vi "Calculate-MSCN x-axis value.vi"(5 "Total number of points in indexed ROI over the full experiment time":i32, 7 "Number of pixels in ROI":i32, 9 "Header Data":T1={"Number of POI"=0, "Number of Miniscans"=0, "Number of Trials"=0, "Number of Cycles "=0, "# Averaged Frames"=0, "Laser power (%)"=0, "Pockels"=0.0, "Acquisition Length (sec)"=0.0, "Fill time (us)"=0.0, "DwellTime (us)"=0.0, "Miniscan Dwell time per pixel (us)"=0.0, "PMT 1"=0.0, "PMT 2"=0.0, "Back Apperture"=0.0, "Zoom"=0.0, "Number of Pixels in Miniscan"=0, "Frame Size"=200, "Field of View"=0.0, "X centre"=0.0, "Y centre"=0.0, "AOL Z"=0.0} {"Frame Size" items=["100X100"=100, "128X128"=128, "200X200"=200, "256X256"=256, "512X512"=512, "1024x1024"=1024, "2048x2048"=2048]; "Back Apperture" format="%#.6g"; "Pockels" format="%#.6g"; "PMT 2" format="%#.6g"; "PMT 1" format="%#.6g"; "Miniscan Dwell time per pixel (us)" format="%#.6g"; "Zoom" format="%#.6g"; "DwellTime (us)" format="%#.6g"; "Acquisition Length (sec)" format="%#.6g"; "Fill time (us)" format="%#.6g"}, 10 "[ROI Time(us)]":dbl[](array[numeric]), 11 "ROI number":i32=1) -> (1 "MSCN X-axis values array (sec)":sgl[](array[numeric]) format="%#.9f")   [LabVIEW 2020]
uses:
  Experiment header interface/Typedefs/Header parameters cluster-Zstack.ctl
  Typedefs/Frame Size.ctl
panel:
  out "Array":i32[](array[numeric])
  # "Zstack header parameters"
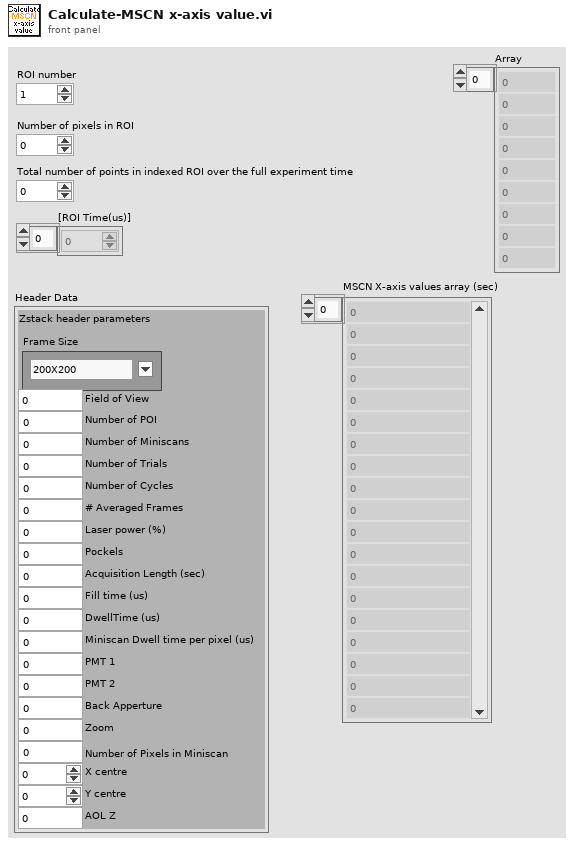
[diagram p1: front panel]
types:
  T1 = typedef "Header parameters cluster-Zstack.ctl" = cluster{"Number of POI":u16, "Number of Miniscans":u16, "Number of Trials":u16, "Number of Cycles ":u16, "# Averaged Frames":u16, "Laser power (%)":u8, "Pockels":dbl, "Acquisition Length (sec)":dbl, "Fill time (us)":dbl, "DwellTime (us)":dbl, "Miniscan Dwell time per pixel (us)":dbl, "PMT 1":dbl, "PMT 2":dbl, "Back Apperture":dbl, "Zoom":dbl, "Number of Pixels in Miniscan":u16, "Frame Size":T2, "Field of View":dbl, "X centre":dbl, "Y centre":dbl, "AOL Z":dbl}
  T2 = typedef "Frame Size.ctl" = u16
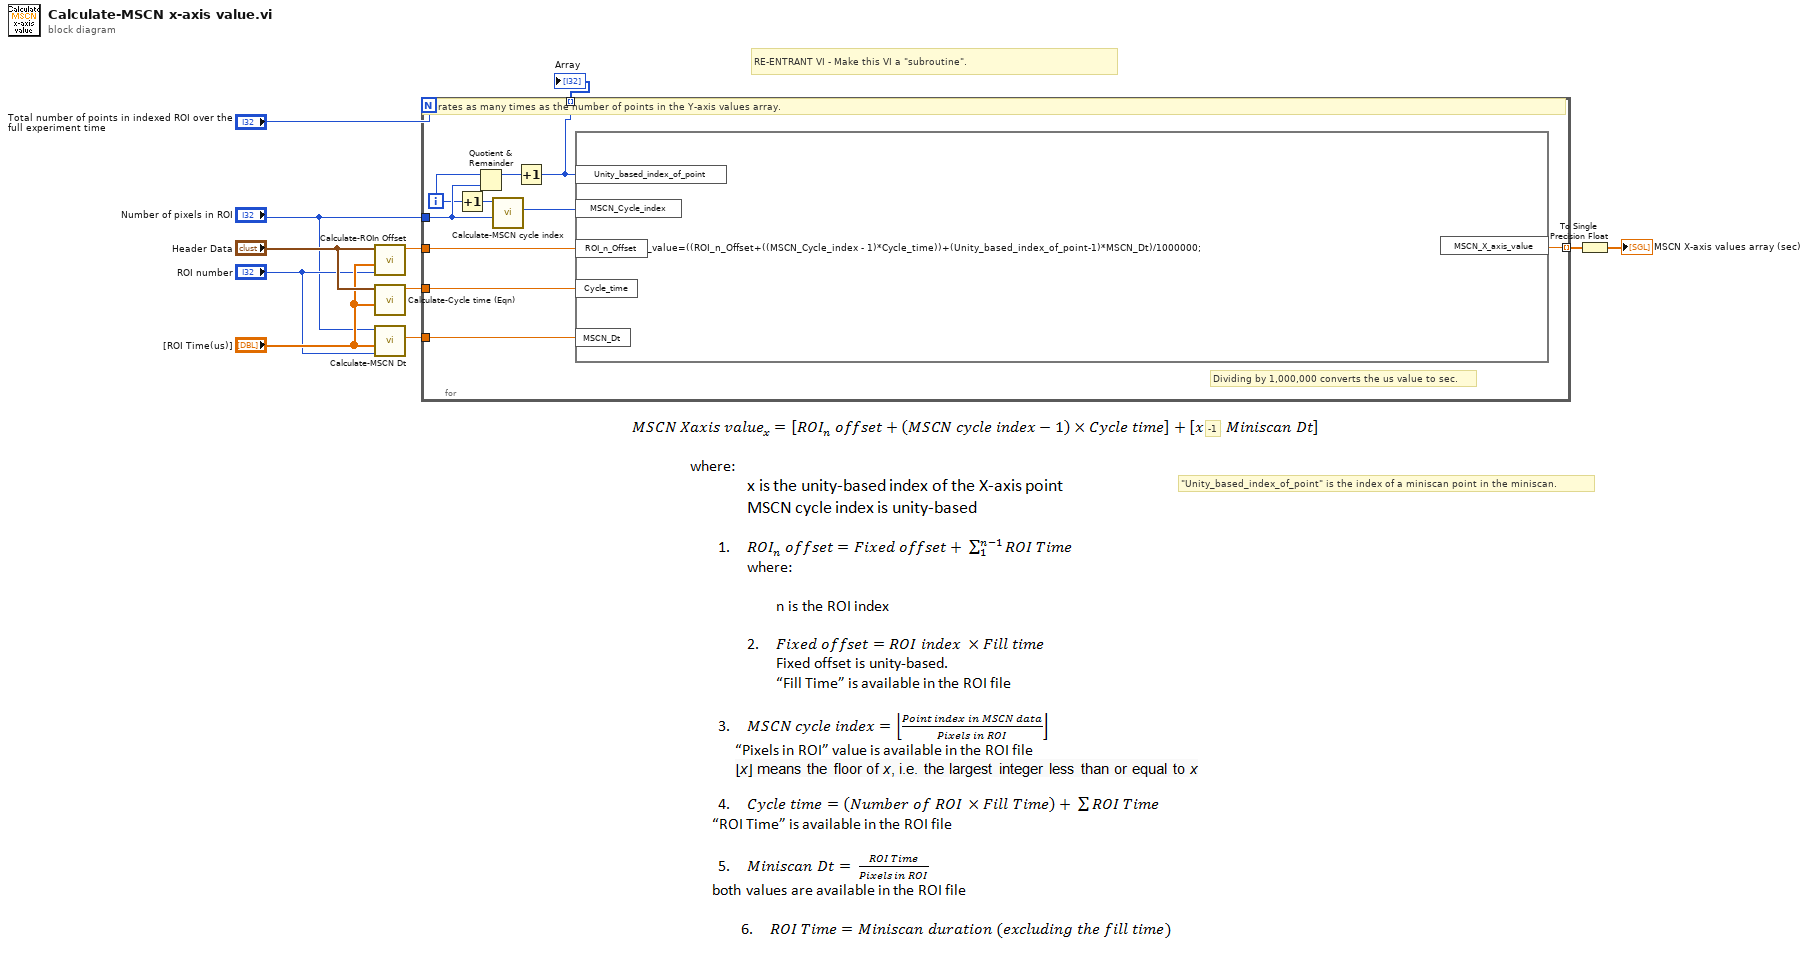
[diagram p0: block diagram]
diagram:
  # "\"Unity_based_index_of_point\" is the index of a miniscan point in the miniscan."
  # "-1"
  # "RE-ENTRANT VI - Make this VI a \"subroutine\"."
  n1 = call "Calculate-ROIn Offset.vi"("ROI number"="ROI number", "[ROI Time(us)]"="[ROI Time(us)]", "Header data"="Header Data") -> ("ROI n Offset (us)"=w9:dbl)  [unwired: 8 in]
  n2 = call "Calculate-Cycle time (Eqn).vi"("[ROI Time (us)]"="[ROI Time(us)]", "Header data"="Header Data") -> ("Cycle Time (us)"=w10:dbl)  [unwired: 9 in]
  n3 = call "Calculate-MSCN Dt.vi"("ROI number"="ROI number", "[ROI Time(us)]"="[ROI Time(us)]", "Number of pixels in ROI"="Number of pixels in ROI") -> ("MSCN Dt"=w6:dbl)  [unwired: 8 in]
  n4 = for {
    N: "Total number of points in indexed ROI over the full experiment time" -> [_]
    tunnel: [w17] -> w3 mode=indexing
    tunnel: w10 -> [w21]
    tunnel: w9 -> [w20]
    tunnel: w6 -> [w19]
    tunnel: "Number of pixels in ROI" -> [w16]
    tunnel: [w12] -> w2 mode=indexing
    i -> [w14]
    # "Dividing by 1,000,000 converts the us value to sec."
    # "Iterates as many times as the number of points in the Y-axis values array."
    n5 = Increment(x=w14) -> (x+1=w15:i32)
    n6 = Quotient & Remainder(x=w14, y=w16) -> (x-y*floor(x/y)=w13:i32)  [unwired: 1 out]
    n7 = call "Calculate-MSCN cycle index.vi"("Number of pixels in ROI"=w16, "Unity based index of miniscan point"=w15) -> ("MSCN Cycle index (unity based)"=w18:i32)  [unwired: 9 in]
    n8 = Increment(x=w13) -> (x+1=w12:i32)
    n9 = formula code="MSCN_X_axis_value=((ROI_n_Offset+((MSCN_Cycle_index - 1)*Cycle_time))+(Unity_based_index_of_point-1)*MSCN_Dt)/1000000;"("MSCN_Cycle_index"=w18, "ROI_n_Offset"=w20, "Cycle_time"=w21, "Unity_based_index_of_point"=w12, "MSCN_Dt"=w19) -> ("MSCN_X_axis_value"=w17:dbl)
  }
  "Array" <- w2
  n10 = To Single Precision Float(number=w3) -> (single precision float=→"MSCN X-axis values array (sec)":sgl[])
